vi "ColorRamp_TS.vi"(9 "max value":i32=100, 10 "value":dbl(slide) scale=0.0..100.0) -> (2 "Color":u32(colorbox)=6618880)   [LabVIEW 2020]
panel:
  out "Array":cluster{"Value":dbl, "Color":u32}[](array[cluster])
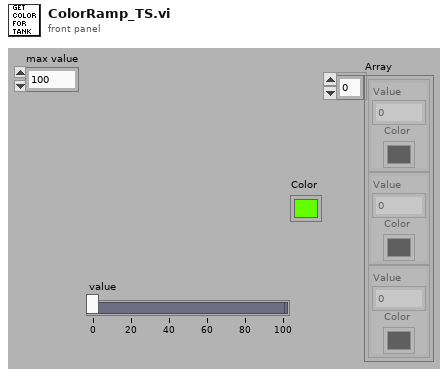
[diagram p1: front panel]
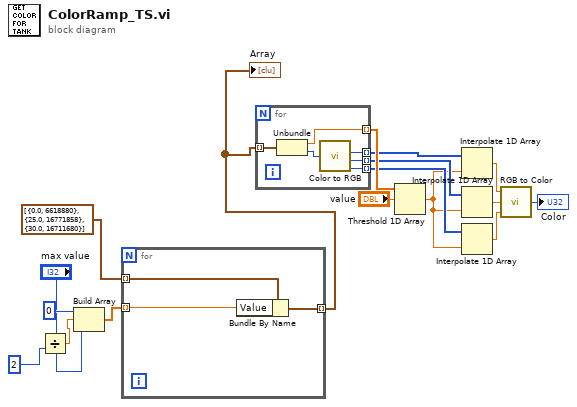
[diagram p0: block diagram]
diagram:
  n1 = Divide(x="max value", y=2) -> (x/y=w4:dbl)
  n2 = Build Array(0, w4, "max value") -> (w2:dbl[])
  n3 = for {
    tunnel: cluster{"Value":dbl, "Color":u32}[] [{"Value"=0.0, "Color"=6618880}, {"Value"=25.0, "Color"=16771858}, {"Value"=30.0, "Color"=16711680}] ("Color Array") -> [w20] mode=indexing
    tunnel: w2 -> [w19] mode=indexing
    tunnel: [w18] -> w1 mode=indexing
    n4 = Bundle By Name(cluster=w20, "Value"=w19) -> (w18:cluster{"Value":dbl, "Color":u32})
  }
  "Array" <- w1
  n5 = for {
    tunnel: w1 -> [w26] mode=indexing
    tunnel: [w24] -> w16 mode=indexing
    tunnel: [w23] -> w15 mode=indexing
    tunnel: [w22] -> w14 mode=indexing
    tunnel: [w21] -> w17 mode=indexing
    n6 = Unbundle(w26) -> ("Value"=w21:dbl, "Color"=w25:u32)
    n7 = call <vilib>:"Color to RGB.vi"("Color"=w25) -> ("R"=w24:u8, "G"=w23:u8, "B"=w22:u8)  [unwired: 1 out]
  }
  n8 = Threshold 1D Array(2:"value", 3:w17) -> (0:w13:dbl)  [unwired: 1 in]
  n9 = Interpolate 1D Array(1:w13, 2:w16) -> (0:w10:dbl)
  n10 = Interpolate 1D Array(1:w13, 2:w15) -> (0:w11:dbl)
  n11 = Interpolate 1D Array(1:w13, 2:w14) -> (0:w12:dbl)
  n12 = call <vilib>:"RGB to Color.vi"("B"=w12, "G"=w11, "R"=w10) -> ("Color"=→"Color":u32)
